vi "projektjki.vi"() -> ()   [LabVIEW 2020]
uses:
  <vilib>/vision/driver/NI_Vision_Acquisition_Software.lvlib
panel:
  out "Informacje":string
  out "Wykryto kamere":bool
  out "?":bool
  out "Mało wody":bool
  out "Dużo wody":bool
  out "Kamera aktywna":bool
  out "Zapis danychh":bool
  in  "Zapis danych":bool
  out "cm^3                                     Tank":dbl(slide) scale=0.0..394.0
  in  "Wl/WYL Kamere":bool
  out "Image":T1(plugin-control)
  in  "Zakoncz":bool
  # "Zbiornik"
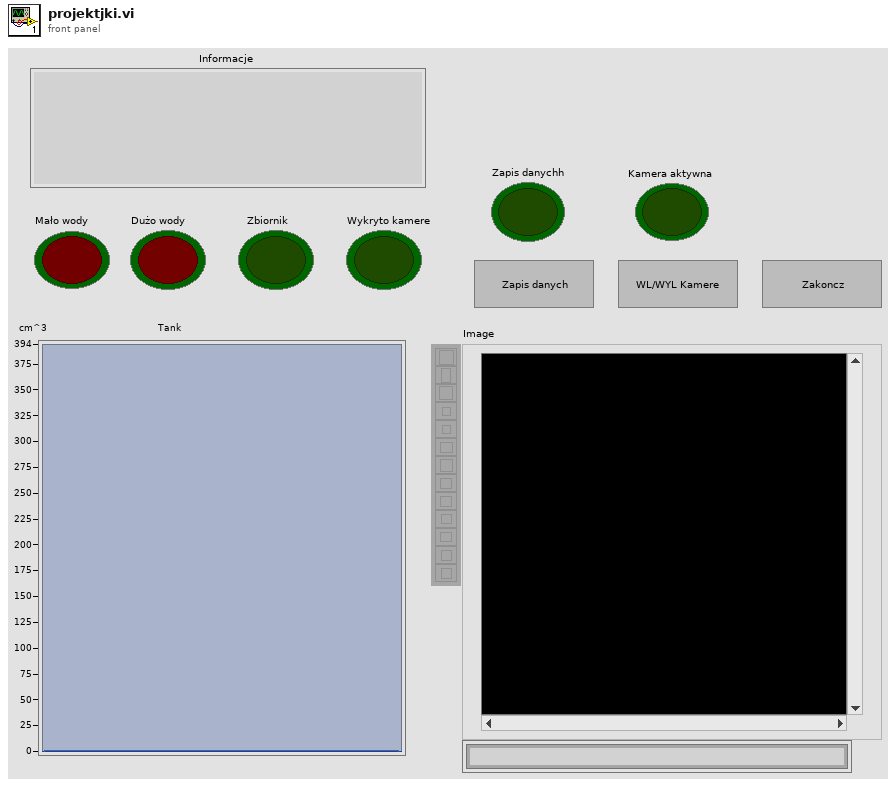
[diagram p1: front panel]
types:
  T1 = typedef "IMAQ Image.ctl" = refnum<image>
  T2 = enum32{"Invalid", "Standard", "Closed", "Hidden", "Minimized", "Maximized"}
  T3 = enum32{"invalid app kind", "Development System", "Run Time System", "Student Edition", "Embedded LabVIEW", "Evaluation", "Custom"}
  T4 = cluster{"Core":cluster{"Current VI Reference":refnum<vi>, "Close Panel on Exit?":bool}, "wykryto kamere":bool, "\nInformacje":string, "Image":T1, "Wylacz kamere":bool, "number of replacements":i32, "historia zbiornika":dbl, "cm^3                                     Tank ":dbl, "Zapis danych":bool, "Mało wody":bool, "Dużo wody":bool, "Wykryto obiekt":bool}
  T5 = cluster{"Current VI Reference":refnum<vi>, "Close Panel on Exit?":bool}
  T6 = cluster{"Point1 (Pixels)":cluster{"X":sgl, "Y":sgl}, "Point2 (Pixels)":cluster{"X":sgl, "Y":sgl}, "Point1 (Real-World)":cluster{"X":sgl, "Y":sgl}, "Point2 (Real-World)":cluster{"X":sgl, "Y":sgl}, "Angle (Pixel)":dbl, "Angle (Real-World)":dbl, "Score":dbl, "Straightness":dbl, "Average SNR (db)":dbl, "Calibration Valid":bool}[]
  T7 = cluster{"Point1 (Pixels)":cluster{"X":sgl, "Y":sgl}, "Point2 (Pixels)":cluster{"X":sgl, "Y":sgl}, "Point1 (Real-World)":cluster{"X":sgl, "Y":sgl}, "Point2 (Real-World)":cluster{"X":sgl, "Y":sgl}, "Angle (Pixel)":dbl, "Angle (Real-World)":dbl, "Score":dbl, "Straightness":dbl, "Average SNR (db)":dbl, "Calibration Valid":bool}
  T8 = cluster{"Type":u32, "Version":u32, "Flags":u32, "SerialNumberHigh":u32, "SerialNumberLow":u32, "BusType":u32, "InterfaceName":string, "VendorName":string, "ModelName":string, "CameraFileName":string, "CameraAttributeURL":string}[]
  T9 = cluster{"Type":u32, "Version":u32, "Flags":u32, "SerialNumberHigh":u32, "SerialNumberLow":u32, "BusType":u32, "InterfaceName":string, "VendorName":string, "ModelName":string, "CameraFileName":string, "CameraAttributeURL":string}
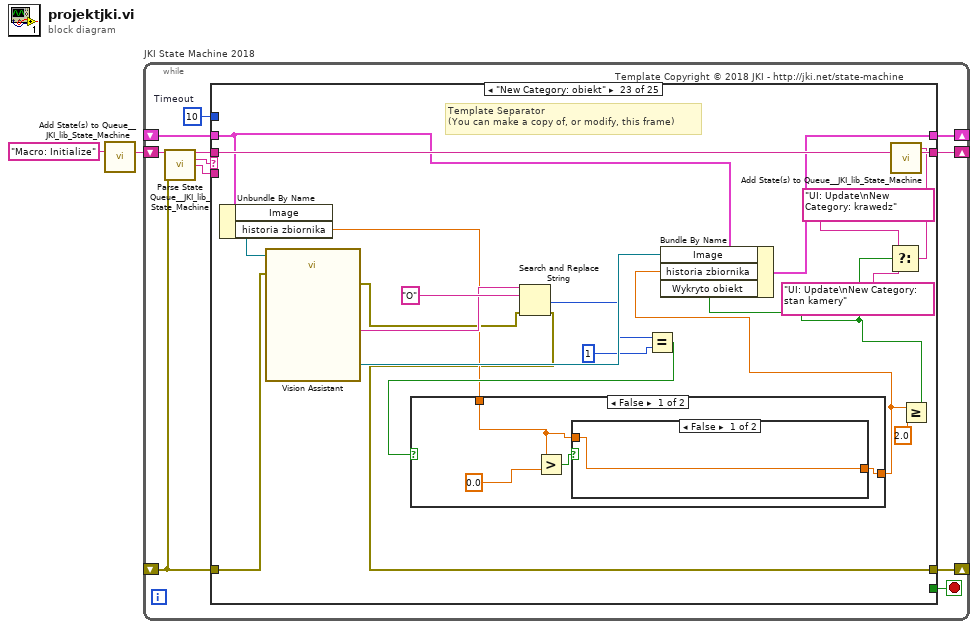
[diagram p0: block diagram]
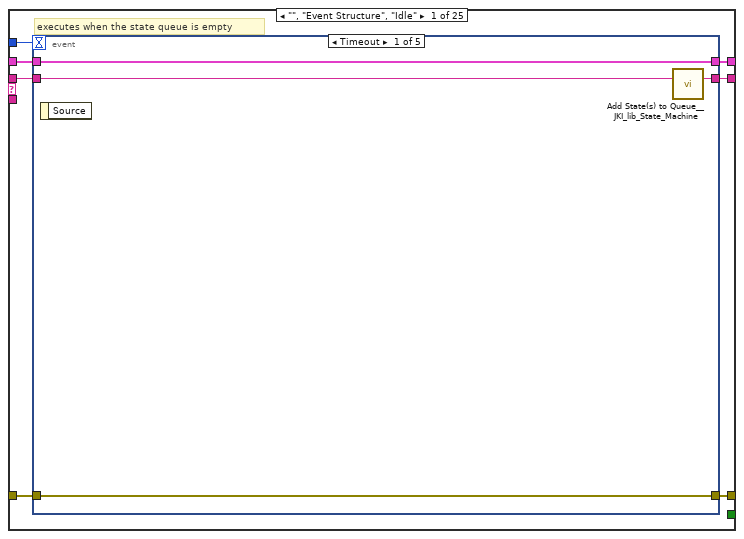
[diagram p2: hidden frame]
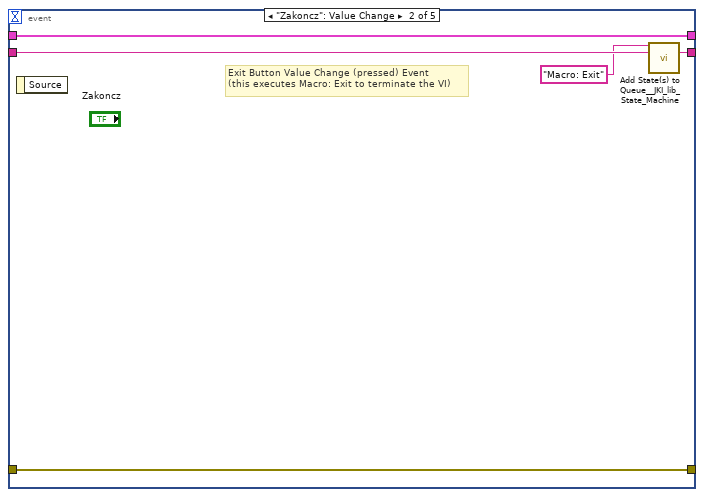
[diagram p3: hidden frame]
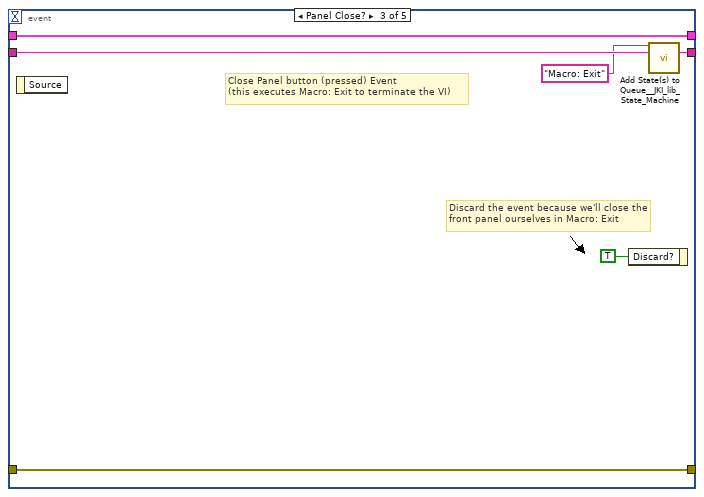
[diagram p4: hidden frame]
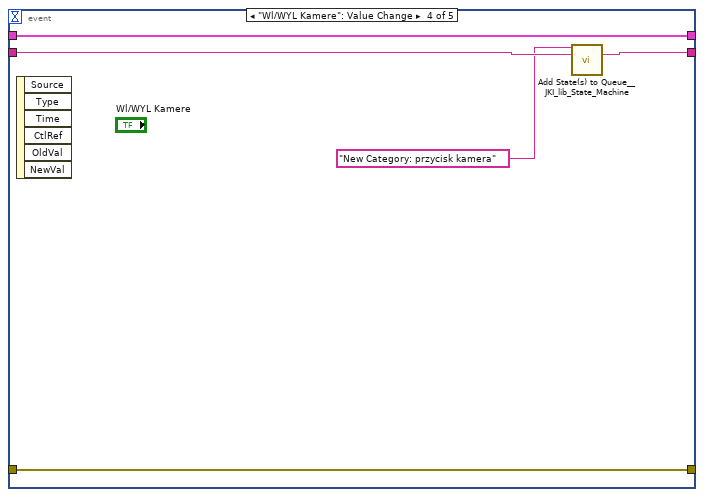
[diagram p5: hidden frame]
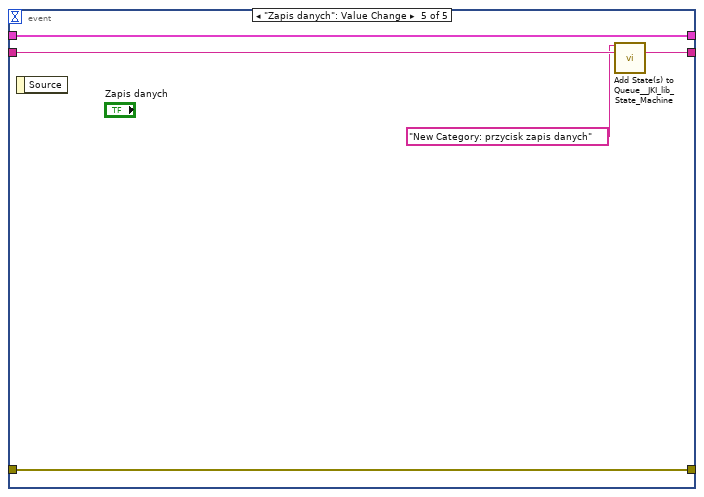
[diagram p6: hidden frame]
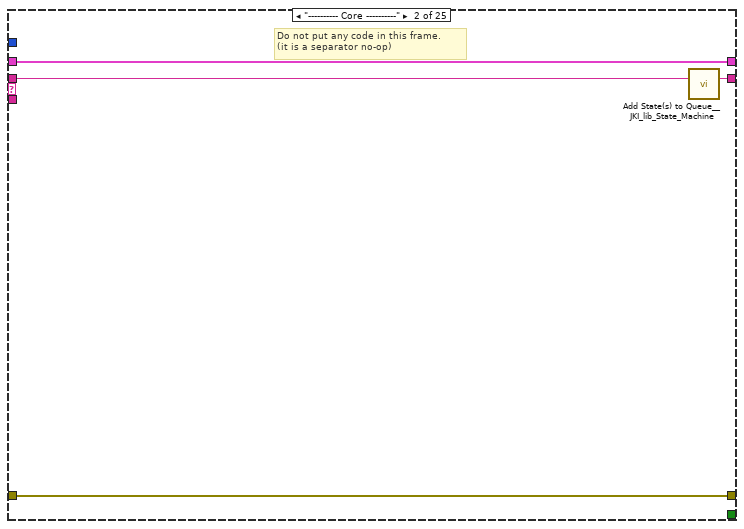
[diagram p7: hidden frame]
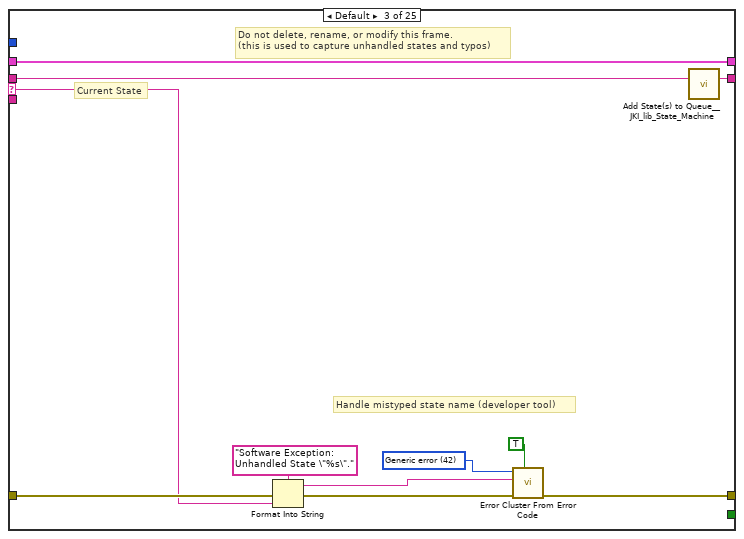
[diagram p8: hidden frame]
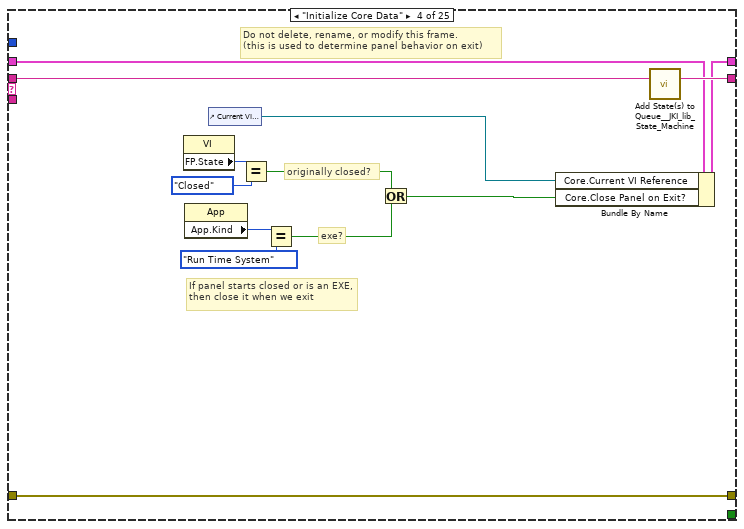
[diagram p9: hidden frame]
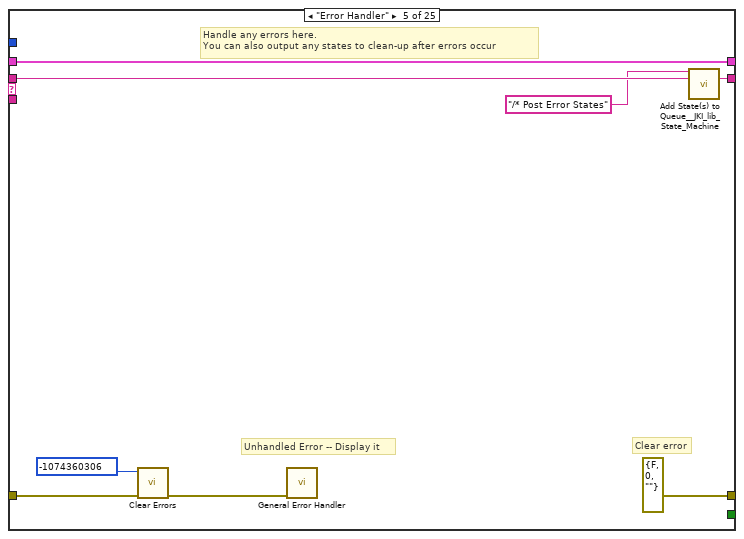
[diagram p10: hidden frame]
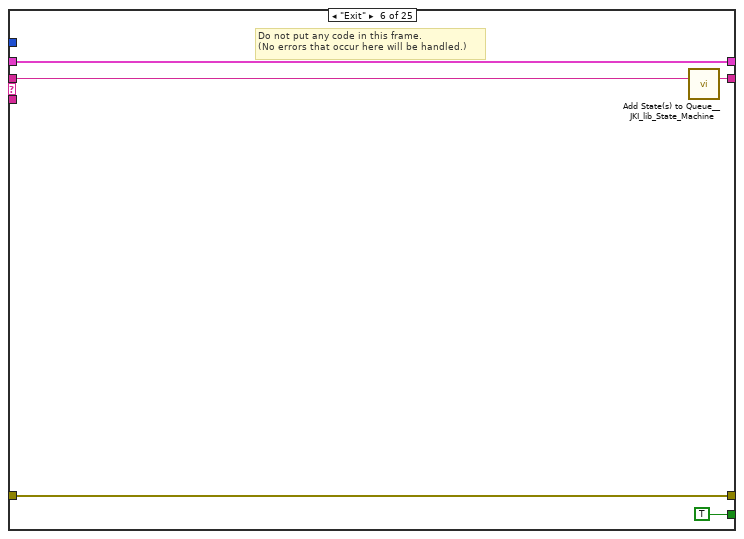
[diagram p11: hidden frame]
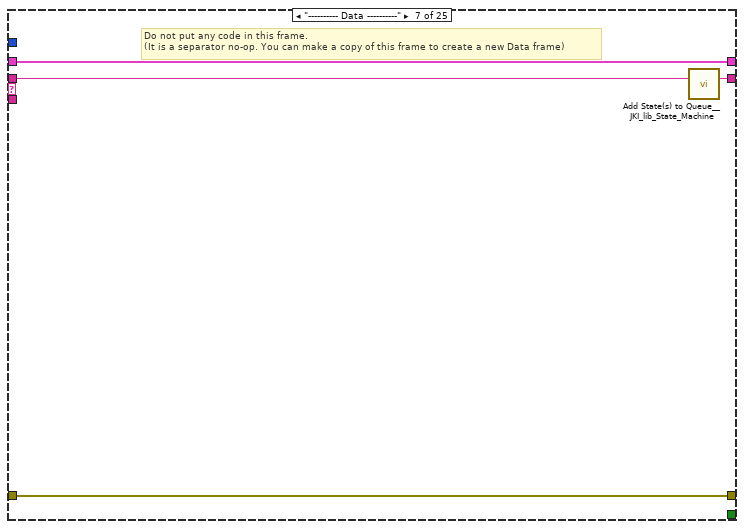
[diagram p12: hidden frame]
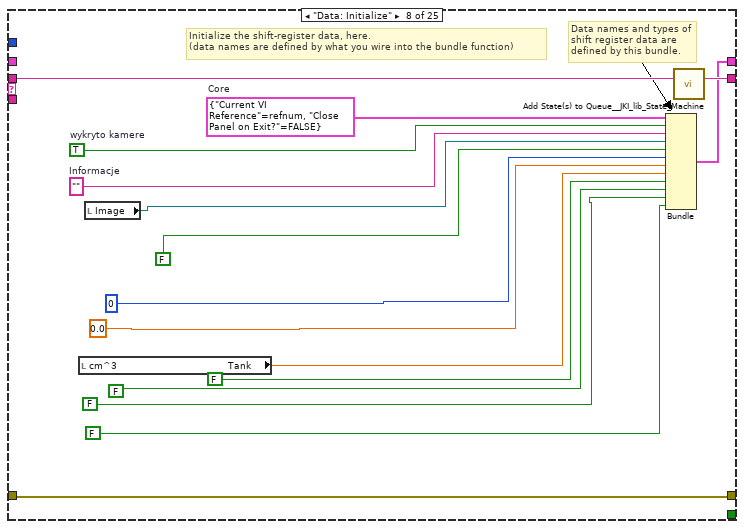
[diagram p13: hidden frame]
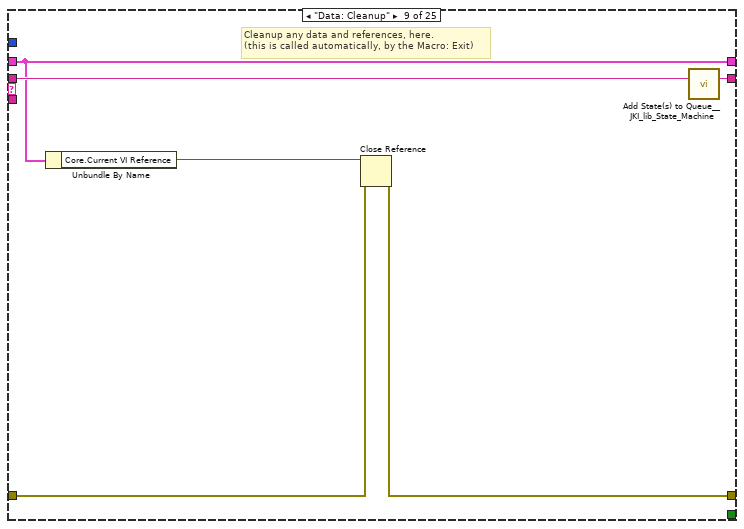
[diagram p14: hidden frame]
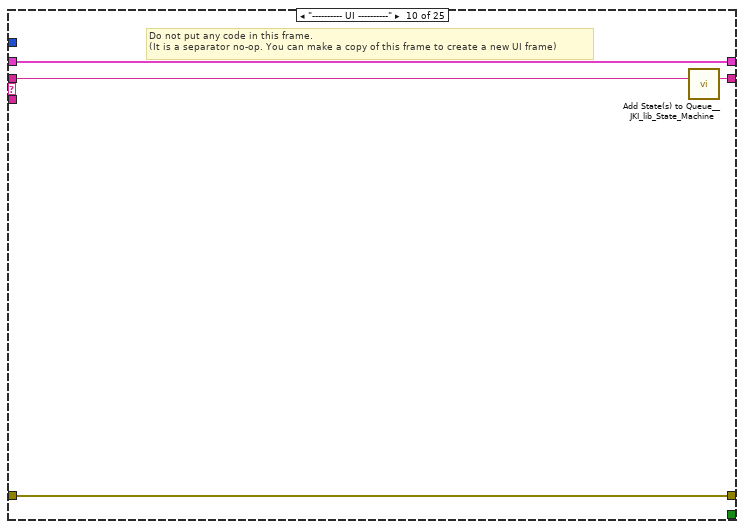
[diagram p15: hidden frame]
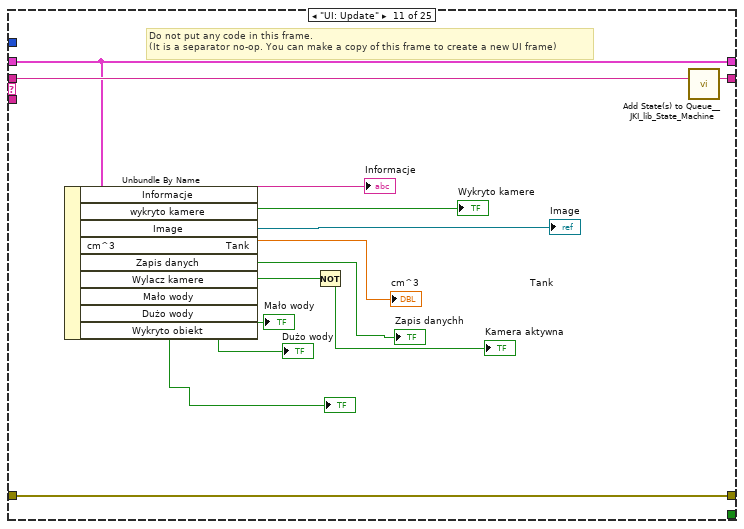
[diagram p16: hidden frame]
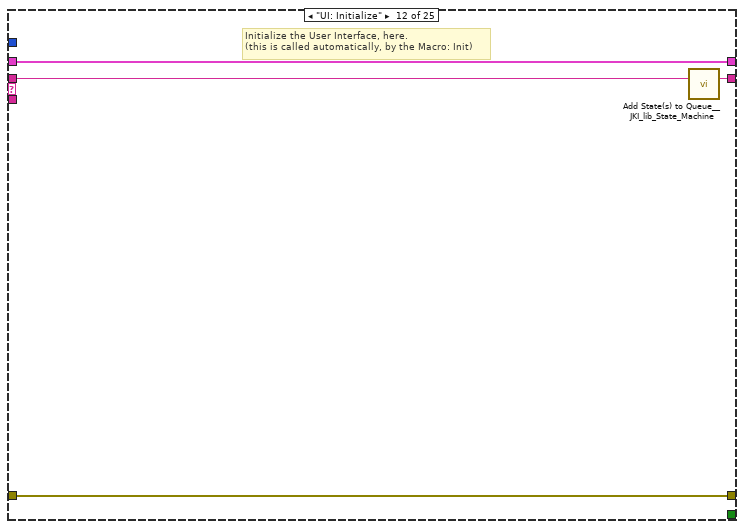
[diagram p17: hidden frame]
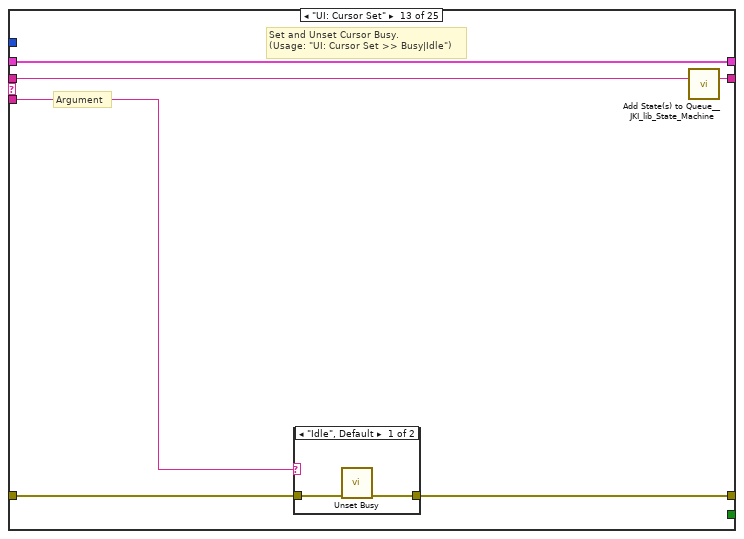
[diagram p18: hidden frame]
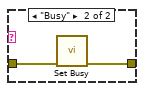
[diagram p19: hidden frame]
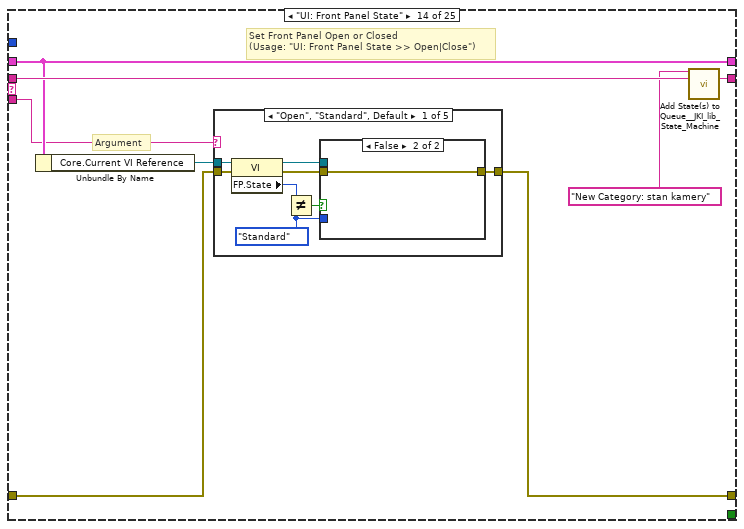
[diagram p20: hidden frame]
diagram:
  n1 = call <vilib>:"Add State(s) to Queue__JKI_lib_State_Machine.vi"("State(s) in (\"\")"="Macro: Initialize") -> ("States Out"=w2:string)  [unwired: 14 in]
  n2 = while "JKI State Machine 2018" {
    shift-right: [w6] -> _
    shift-left: _ -> [w5]
    shift-right: [w9] -> _
    shift-left: _ -> [w3]
    shift-right: [w8] -> _
    shift-left: w2 -> [w10]
    stop <- w7 stop-if-true
    w4 = 10  # Timeout
    # "Template Copyright © 2018 JKI - http://jki.net/state-machine"
    n3 = call <vilib>:"Parse State Queue__JKI_lib_State_Machine.vi"("State Queue"=w10, "Error In (no error)"=w3) -> ("Remaining States"=w12:string, "Current State"=w13:string, "Arguments"=w11:string)  [unwired: 11 in]
    n4 = case shown="\"New Category: obiekt\"" w13 {
      selector: w13 -> [_ _ w50 _ _ _ _ _ _ _ _ _ _ _ _ _ _ _ _ _ _ _ _ _ _]
      tunnel: w12 -> [w20 w49 w54 w73 w81 w86 w90 w106 w112 w116 w130 w134 w140 w152 w221 w231 w236 w240 w250 w257 w270 w288 w324 w353 w374]
      tunnel: w11 -> [_ _ _ _ _ _ _ _ _ _ _ _ w135 w146 _ _ _ _ _ _ _ _ _ _ _]
      tunnel: w5 -> [w18 w46 w52 w66 w78 w84 w87 _ w107 w113 w127 w132 w138 w148 w218 w228 w233 w237 w247 w253 w260 w280 w320 w349 w360]
      tunnel: [w17 w47 w56 w70 errorcluster {"status"=FALSE, "code"=0, "source"=""} ("error out") w83 w88 w103 w108 w114 w128 w131 w136 w149 w219 w229 w234 w238 w248 w255 w265 w278 w304 w341 w371] -> w9
      tunnel: w3 -> [w16 w47 w55 w70 w74 w83 w88 w103 w109 w114 w128 w131 w137 w150 w219 w229 w234 w238 w248 w255 w264 w277 w307 w343 w370]
      tunnel: [w19 w48 w53 w72 w80 w85 w89 w105 w111 w115 w129 w133 w139 w151 w220 w230 w235 w239 w249 w256 w269 w287 w323 w352 w373] -> w8
      tunnel: [_ _ _ _ _ TRUE _ _ _ _ _ _ _ _ _ _ _ _ _ _ _ _ _ _ _] -> w7
      tunnel: [w15 w46 w52 w71 w78 w84 w87 w104 w107 w113 w127 w132 w138 w148 w218 w228 w233 w237 w243 w254 w261 w281 w321 w351 w361] -> w6
      tunnel: w4 -> [w14 _ _ _ _ _ _ _ _ _ _ _ _ _ _ _ _ _ _ _ _ _ _ _ _]
      frame "", "Event Structure", "Idle" {
        # "executes when the state queue is empty"
        n5 = event shown="[0] Timeout" {
          selector: _ -> [_ _ _ _ _]
          dyn-events: _ -> [_ _ _ _ _]
          timeout: w14 -> [_ _ _ _ _]
          tunnel: w20 -> [w24 w29 w35 w37 w43]
          tunnel: [w23 w28 w34 w38 w44] -> w19
          tunnel: w18 -> [w21 w26 w32 w40 w45]
          tunnel: [w22 w27 w33 w39 w41] -> w17
          tunnel: w16 -> [w22 w27 w33 w39 w41]
          tunnel: [w21 w26 w32 w40 w45] -> w15
          event Timeout {
            n6 = event-data() -> ()  [unwired: 1 in, 1 out]
            n7 = call <vilib>:"Add State(s) to Queue__JKI_lib_State_Machine.vi"("State(s) in (\"\")"=w24) -> ("States Out"=w23:string)  [unwired: 14 in]
          }
          event "Zakoncz": Value Change {
            # "Exit Button Value Change (pressed) Event\n(this executes Macro: Exit to terminate the VI)"
            n8 = event-data() -> ()  [unwired: 1 in, 1 out]
            n9 = call <vilib>:"Add State(s) to Queue__JKI_lib_State_Machine.vi"("State(s) in Front (\"\")"="Macro: Exit", "State(s) in (\"\")"=w29) -> ("States Out"=w28:string)  [unwired: 13 in]
          }
          event Panel Close? {
            # "Discard the event because we'll close the front panel ourselves in Macro: Exit"
            # "Close Panel button (pressed) Event\n(this executes Macro: Exit to terminate the VI)"
            n10 = event-data() -> ()  [unwired: 1 in, 1 out]
            n11 = event-data ("Event Filter Node")("Discard?"=TRUE) -> ()  [unwired: 1 in, 1 out]
            n12 = call <vilib>:"Add State(s) to Queue__JKI_lib_State_Machine.vi"("State(s) in Front (\"\")"="Macro: Exit", "State(s) in (\"\")"=w35) -> ("States Out"=w34:string)  [unwired: 13 in]
          }
          event "Wl/WYL Kamere": Value Change {
            n13 = event-data() -> ()  [unwired: 1 in, 6 out]
            n14 = call <vilib>:"Add State(s) to Queue__JKI_lib_State_Machine.vi"("State(s) in Front (\"\")"="New Category: przycisk kamera" ("State(s) in Front (\"\")"), "State(s) in (\"\")"=w37) -> ("States Out"=w38:string)  [unwired: 13 in]
          }
          event "Zapis danych": Value Change {
            n15 = event-data() -> ()  [unwired: 1 in, 1 out]
            n16 = call <vilib>:"Add State(s) to Queue__JKI_lib_State_Machine.vi"("State(s) in Front (\"\")"="New Category: przycisk zapis danych" ("State(s) in Front (\"\")"), "State(s) in (\"\")"=w43) -> ("States Out"=w44:string)  [unwired: 13 in]
          }
        }
      }
      frame "---------- Core ----------" {
        # "Do not put any code in this frame.\n(it is a separator no-op)"
        n17 = call <vilib>:"Add State(s) to Queue__JKI_lib_State_Machine.vi"("State(s) in (\"\")"=w49) -> ("States Out"=w48:string)  [unwired: 14 in]
      }
      frame Default {
        w59 = 42 items=["No error", "Argument error", "Memory is full", "Out of zone", "End of file", "File already open", "Generic file I/O error", "File not found", "File permission error", "Disk is full", "Duplicate path", "Too many files open", "System feature not enabled", "Resource file not found", "Cannot add resource", "Resource not found", "Image not found", "Image memory error", "Pen does not exist", "Config type invalid", "Config token not found", "Config parse error", "Config memory error", "Bad external code format", "Bad external code offset", "External code not present", "Null window", "Destroy window error", "Null menu", "Print aborted", "Bad print record", "Print driver error", "Windows error during printing", "Memory error during printing", "Print dialog error", "Generic print error", "Invalid device refnum", "Device not found", "Device parameter error", "Device unit error", "Cannot open device", "Device call aborted", "Generic error", "Cancelled by user", "Object ID too low", "Object ID too high", "Object not in heap", "Unknown heap", "Unknown object (invalid DefProc)", "Unknown object (DefProc not in table)", "Message out of range", "Invalid (null) method", "Unknown message", "Manager call not supported", "Bad address", "Network operation in progress", "Network operation timed out", "Connection is busy", "Network attribute not supported", "Network error", "Address in use", "System out of memory", "Connection aborted", "Connection refused", "Not connected", "Already connected", "Connection closed", "Initialization error (interapplication manager)", "Bad occurrence", "Wait on unbound occurrence handler", "Occurrence queue overflow", "Datalog type conflict", "Unused", "Unrecognized type (interapplication manager)", "Memory corrupt", "Failed to make temporary DLL", "Old CIN version", "Drag socket not found", "Failed to load drop-object", "Failed to register OLE object", "Failed to release OLE object", "Format specifier type mismatch", "Unknown format specifier", "Too few format specifiers", "Too many format specifiers", "Scan failed", "Newer CIN version", "Error converting to variant", "Runtime menu error", "Password tampered", "Variant attribute not found", "Incompatible variant data type", "Event data is not available", "Event Store is not present", "Occurrence is not found", "Event Queue is not created", "Event info is not available", "Refnum passed is NULL", "Error retrieving Class GUID", "Error retrieving CoClass GUID", "Error retrieving TypeLib GUID.", "Bad built application magic bytes.", "Specific driver is different from the specific driver associated with the Logical Name.", "There is no session opened to the class driver.", "Max Error", "MAX - Error with config objects", "MAX - Error loading configuration", "MAX - Group not supported"]
        # "Current State"
        # "Do not delete, rename, or modify this frame.\n(this is used to capture unhandled states and typos)"
        # "Handle mistyped state name (developer tool)"
        n18 = Format Into String(format string="Software Exception: Unhandled State \"%s\"." ("message"), error in=w55, w50) -> (resulting string=w58:string, error out=w57:errorcluster)  [unwired: 1 in]
        n19 = call <vilib>:"Error Cluster From Error Code.vi"("show call chain? (False)"=TRUE, "error in (no error)"=w57, "error message (\"\")"=w58, "error code (0)"=w59) -> ("error out"=w56:errorcluster)  [unwired: 5 in]
        n20 = call <vilib>:"Add State(s) to Queue__JKI_lib_State_Machine.vi"("State(s) in (\"\")"=w54) -> ("States Out"=w53:string)  [unwired: 14 in]
      }
      frame "Initialize Core Data" {
        # "Do not delete, rename, or modify this frame.\n(this is used to determine panel behavior on exit)"
        # "originally closed?"
        # "exe?"
        # "If panel starts closed or is an EXE, then close it when we exit"
        n21 = property on="Property Node" class="VI"() -> ("FP.State"=w63:T2)  [unwired: 2 in, 2 out]
        n22 = property on="Property Node" class="App"() -> ("App.Kind"=w69:T3)  [unwired: 2 in, 2 out]
        n23 = control-ref of="Current VI Reference"() -> (w64:refnum<vi>)
        n24 = Equal?(x=w63, y=T2."Closed" ("Front Panel Window:State")) -> (x = y?=w61:bool)
        n25 = Equal?(x=w69, y=T3."Run Time System" ("Application:Kind")) -> (x = y?=w67:bool)
        n26 = Or(x=w61, y=w67) -> (x .or. y?=w65:bool)
        n27 = Bundle By Name(cluster=w66, "Core.Current VI Reference"=w64, "Core.Close Panel on Exit?"=w65) -> (w71:T4)
        n28 = call <vilib>:"Add State(s) to Queue__JKI_lib_State_Machine.vi"("State(s) in (\"\")"=w73) -> ("States Out"=w72:string)  [unwired: 14 in]
      }
      frame "Error Handler" {
        # "Unhandled Error -- Display it"
        # "Handle any errors here.\nYou can also output any states to clean-up after errors occur"
        # "Clear error"
        n29 = call <vilib>:"Clear Errors.vi"("error in (no error)"=w74, "specific error code to clear (0: all)"=-1074360306) -> ("error out"=w75:errorcluster)  [unwired: 4 in, 1 out]
        n30 = call <vilib>:"General Error Handler.vi"("error in (no error)"=w75) -> ()  [unwired: 10 in, 5 out]
        n31 = call <vilib>:"Add State(s) to Queue__JKI_lib_State_Machine.vi"("State(s) in Front (\"\")"="/* Post Error States", "State(s) in (\"\")"=w81) -> ("States Out"=w80:string)  [unwired: 13 in]
      }
      frame "Exit" {
        # "Do not put any code in this frame.\n(No errors that occur here will be handled.)"
        n32 = call <vilib>:"Add State(s) to Queue__JKI_lib_State_Machine.vi"("State(s) in (\"\")"=w86) -> ("States Out"=w85:string)  [unwired: 14 in]
      }
      frame "---------- Data ----------" {
        # "Do not put any code in this frame.\n(It is a separator no-op. You can make a copy of this frame to create a new Data frame)"
        n33 = call <vilib>:"Add State(s) to Queue__JKI_lib_State_Machine.vi"("State(s) in (\"\")"=w90) -> ("States Out"=w89:string)  [unwired: 14 in]
      }
      frame "Data: Initialize" {
        w100 = T5 {"Current VI Reference"=refnum, "Close Panel on Exit?"=FALSE}  # Core
        w102 = TRUE  # wykryto kamere
        w101 = ""  # Informacje
        # "Data names and types of shift register data are defined by this bundle."
        # "Initialize the shift-register data, here.\n(data names are defined by what you wire into the bundle function)"
        n34 = local read "cm^3                                     Tank"() -> (w98:dbl)
        n35 = local read "Image"() -> (w91:T1)
        n36 = Bundle("Core"=w100, "wykryto kamere"=w102, "Informacje"=w101, "Image"=w91, "Wylacz kamere"=FALSE, "number of replacements"=0, "historia zbiornika"=0.0, "cm^3                                     Tank"=w98, "Zapis danych"=FALSE, "Mało wody"=FALSE, "Dużo wody"=FALSE, "Wykryto obiekt"=FALSE) -> (w104:T4)  [unwired: 1 in]
        n37 = call <vilib>:"Add State(s) to Queue__JKI_lib_State_Machine.vi"("State(s) in (\"\")"=w106) -> ("States Out"=w105:string)  [unwired: 14 in]
      }
      frame "Data: Cleanup" {
        # "Cleanup any data and references, here.\n(this is called automatically, by the Macro: Exit)"
        n38 = Unbundle By Name(w107) -> ("Core.Current VI Reference"=w110:refnum<vi>)
        n39 = Close Reference(reference=w110, error in (no error)=w109) -> (error out=w108:errorcluster)
        n40 = call <vilib>:"Add State(s) to Queue__JKI_lib_State_Machine.vi"("State(s) in (\"\")"=w112) -> ("States Out"=w111:string)  [unwired: 14 in]
      }
      frame "---------- UI ----------" {
        # "Do not put any code in this frame.\n(It is a separator no-op. You can make a copy of this frame to create a new UI frame)"
        n41 = call <vilib>:"Add State(s) to Queue__JKI_lib_State_Machine.vi"("State(s) in (\"\")"=w116) -> ("States Out"=w115:string)  [unwired: 14 in]
      }
      frame "UI: Update" {
        # "Do not put any code in this frame.\n(It is a separator no-op. You can make a copy of this frame to create a new UI frame)"
        n42 = Unbundle By Name(w127) -> ("Informacje"=→"Informacje":string, "wykryto kamere"=→"Wykryto kamere":bool, "Image"=→"Image":T1, "cm^3                                     Tank"=→"cm^3                                     Tank":dbl, "Zapis danych"=→"Zapis danychh":bool, "Wylacz kamere"=w123:bool, "Mało wody"=→"Mało wody":bool, "Dużo wody"=→"Dużo wody":bool, "Wykryto obiekt"=→"?":bool)
        n43 = Not(x=w123) -> (.not. x?=→"Kamera aktywna":bool)
        n44 = call <vilib>:"Add State(s) to Queue__JKI_lib_State_Machine.vi"("State(s) in (\"\")"=w130) -> ("States Out"=w129:string)  [unwired: 14 in]
      }
      frame "UI: Initialize" {
        # "Initialize the User Interface, here.\n(this is called automatically, by the Macro: Init)"
        n45 = call <vilib>:"Add State(s) to Queue__JKI_lib_State_Machine.vi"("State(s) in (\"\")"=w134) -> ("States Out"=w133:string)  [unwired: 14 in]
      }
      frame "UI: Cursor Set" {
        # "Argument"
        # "Set and Unset Cursor Busy.\n(Usage: \"UI: Cursor Set >> Busy|Idle\")"
        n46 = case shown="\"Idle\", Default" w135 {
          tunnel: w137 -> [w142 w144]
          tunnel: [w141 w143] -> w136
          frame "Idle", Default {
            n47 = call <vilib>:"Unset Busy.vi"("error in (no error)"=w142) -> ("error out"=w141:errorcluster)  [unwired: 10 in]
          }
          frame "Busy" {
            n48 = call <vilib>:"Set Busy.vi"("error in (no error)"=w144) -> ("error out"=w143:errorcluster)  [unwired: 9 in, 1 out]
          }
        }
        n49 = call <vilib>:"Add State(s) to Queue__JKI_lib_State_Machine.vi"("State(s) in (\"\")"=w140) -> ("States Out"=w139:string)  [unwired: 14 in]
      }
      frame "UI: Front Panel State" {
        # "Argument"
        # "Set Front Panel Open or Closed\n(Usage: \"UI: Front Panel State >> Open|Close\")"
        n50 = Unbundle By Name(w148) -> ("Core.Current VI Reference"=w147:refnum<vi>)
        n51 = case shown="\"Open\", \"Standard\", Default" w146 {
          tunnel: w150 -> [w158 w173 w184 w197 w210]
          tunnel: [w160 w174 w186 w199 w212] -> w149
          tunnel: w147 -> [w159 w171 w185 w198 w211]
          frame "Open", "Standard", Default {
            w153 = T2."Standard" ("State")
            n52 = property on="Property Node" class="VI"(reference=w159, error in=w158) -> (reference out=w156:refnum<vi>, error out=w157:errorcluster, "FP.State"=w155:T2)
            n53 = Not Equal?(x=w155, y=w153) -> (x != y?=w154:bool)
            n54 = case shown="False" w154 {
              tunnel: [w164 w166] -> w160
              tunnel: w157 -> [w163 w166]
              tunnel: w156 -> [w162 _]
              tunnel: w153 -> [w161 _]
              frame True {
                n55 = invoke on="Invoke Node" class="VI" method="FP.Open"(reference=w162, error in=w163, "Activate"=TRUE, "State"=w161) -> (error out=w164:errorcluster)  [unwired: 1 in, 4 out]
              }
              frame False {
              }
            }
          }
          frame "Close", "Closed" {
            n56 = property on="Property Node" class="VI"(reference=w171, error in=w173) -> (reference out=w170:refnum<vi>, error out=w172:errorcluster, "FP.State"=w168:T2)
            n57 = Not Equal?(x=w168, y=T2."Closed" ("Front Panel Window:State")) -> (x != y?=w167:bool)
            n58 = case shown="True" w167 {
              tunnel: [w175 w178] -> w174
              tunnel: w172 -> [w175 w177]
              tunnel: w170 -> [_ w176]
              frame False {
              }
              frame True {
                n59 = invoke on="Invoke Node" class="VI" method="FP.Close"(reference=w176, error in=w177) -> (error out=w178:errorcluster)  [unwired: 1 in, 2 out]
              }
            }
          }
          frame "Hidden", "Hide" {
            w179 = T2."Hidden" ("State")
            n60 = property on="Property Node" class="VI"(reference=w185, error in=w184) -> (reference out=w182:refnum<vi>, error out=w183:errorcluster, "FP.State"=w181:T2)
            n61 = Not Equal?(x=w181, y=w179) -> (x != y?=w180:bool)
            n62 = case shown="True" w180 {
              tunnel: [w190 w191] -> w186
              tunnel: w183 -> [w189 w191]
              tunnel: w182 -> [w188 _]
              tunnel: w179 -> [w187 _]
              frame True {
                n63 = invoke on="Invoke Node" class="VI" method="FP.Open"(reference=w188, error in=w189, "State"=w187) -> (error out=w190:errorcluster)  [unwired: 2 in, 4 out]
              }
              frame False {
              }
            }
          }
          frame "Minimize", "Minimized" {
            w192 = T2."Minimized" ("State")
            n64 = property on="Property Node" class="VI"(reference=w198, error in=w197) -> (reference out=w195:refnum<vi>, error out=w196:errorcluster, "FP.State"=w194:T2)
            n65 = Not Equal?(x=w194, y=w192) -> (x != y?=w193:bool)
            n66 = case shown="True" w193 {
              tunnel: [w203 w204] -> w199
              tunnel: w196 -> [w202 w204]
              tunnel: w195 -> [w201 _]
              tunnel: w192 -> [w200 _]
              frame True {
                n67 = invoke on="Invoke Node" class="VI" method="FP.Open"(reference=w201, error in=w202, "State"=w200) -> (error out=w203:errorcluster)  [unwired: 2 in, 4 out]
              }
              frame False {
              }
            }
          }
          frame "Maximize", "Maximized" {
            w205 = T2."Maximized" ("State")
            n68 = property on="Property Node" class="VI"(reference=w211, error in=w210) -> (reference out=w208:refnum<vi>, error out=w209:errorcluster, "FP.State"=w207:T2)
            n69 = Not Equal?(x=w207, y=w205) -> (x != y?=w206:bool)
            n70 = case shown="True" w206 {
              tunnel: [w216 w217] -> w212
              tunnel: w209 -> [w215 w217]
              tunnel: w208 -> [w214 _]
              tunnel: w205 -> [w213 _]
              frame True {
                n71 = invoke on="Invoke Node" class="VI" method="FP.Open"(reference=w214, error in=w215, "State"=w213) -> (error out=w216:errorcluster)  [unwired: 2 in, 4 out]
              }
              frame False {
              }
            }
          }
        }
        n72 = call <vilib>:"Add State(s) to Queue__JKI_lib_State_Machine.vi"("State(s) in Front (\"\")"="New Category: stan kamery" ("State(s) in Front (\"\")"), "State(s) in (\"\")"=w152) -> ("States Out"=w151:string)  [unwired: 13 in]
      }
      frame "---------- Macro ----------" {
        # "Do not put any code in this frame.\n(It is a separator no-op. You can make a copy of this frame to create a new Macro frame)"
        n73 = call <vilib>:"Add State(s) to Queue__JKI_lib_State_Machine.vi"("State(s) in (\"\")"=w221) -> ("States Out"=w220:string)  [unwired: 14 in]
      }
      frame "Macro: Exit" {
        # "Exit Macro\n(This is called once, when the VI exits)"
        n74 = Unbundle By Name(w228) -> ("Core.Close Panel on Exit?"=w227:bool)
        n75 = Select(t="UI: Front Panel State >> Close", s=w227, f="" ("Empty String Constant")) -> (s? t:f=w224:string)
        n76 = call <vilib>:"Add State(s) to Queue__JKI_lib_State_Machine.vi"("State(s) in (\"\")"=w224, "State(s) at Back (\"\")"="Data: Cleanup\nExit") -> ("States Out"=w222:string)  [unwired: 13 in]
        n77 = call <vilib>:"Add State(s) to Queue__JKI_lib_State_Machine.vi"("State(s) in Front (\"\")"=w222, "State(s) in (\"\")"=w231) -> ("States Out"=w230:string)  [unwired: 13 in]
      }
      frame "Macro: Initialize" {
        w232 = "Data: Initialize\nInitialize Core Data\nUI: Initialize\nUI: Front Panel State >> Open"  # Data: Initialize Initialize Core Data UI: Initialize UI: Front Panel State >> Open
        # "Initialization Macro\n(This is called once, when the VI starts)"
        n78 = call <vilib>:"Add State(s) to Queue__JKI_lib_State_Machine.vi"("State(s) in Front (\"\")"=w232, "State(s) in (\"\")"=w236) -> ("States Out"=w235:string)  [unwired: 13 in]
      }
      frame "---------- New Category ----------" {
        # "Template Separator\n(You can make a copy of, or modify, this frame)"
        n79 = call <vilib>:"Add State(s) to Queue__JKI_lib_State_Machine.vi"("State(s) in (\"\")"=w240) -> ("States Out"=w239:string)  [unwired: 14 in]
      }
      frame "New Category: przycisk kamera" {
        # "Template Separator\n(You can make a copy of, or modify, this frame)"
        n80 = Unbundle By Name(w247) -> ("Wylacz kamere"=w246:bool)
        n81 = Not(x=w246) -> (.not. x?=w242:bool)
        n82 = Bundle By Name(cluster=w247, "Wylacz kamere"=w242) -> (w243:T4)
        n83 = Select(t="UI: Update\nNew Category: stan kamery" ("State(s) in Front (\"\")"), s=w242, f="UI: Update\nNew Category: stan kamery") -> (s? t:f=w245:string)
        n84 = call <vilib>:"Add State(s) to Queue__JKI_lib_State_Machine.vi"("State(s) in Front (\"\")"=w245, "State(s) in (\"\")"=w250) -> ("States Out"=w249:string)  [unwired: 13 in]
      }
      frame "New Category: przycisk zapis danych" {
        # "Template Separator\n(You can make a copy of, or modify, this frame)"
        n85 = Unbundle By Name(w253) -> ("Zapis danych"=w252:bool)
        n86 = Not(x=w252) -> (.not. x?=w251:bool)
        n87 = Bundle By Name(cluster=w253, "Zapis danych"=w251) -> (w254:T4)
        n88 = call <vilib>:"Add State(s) to Queue__JKI_lib_State_Machine.vi"("State(s) in (\"\")"=w257) -> ("States Out"=w256:string)  [unwired: 14 in]
      }
      frame "New Category: zapis danych" {
        # "Template Separator\n(You can make a copy of, or modify, this frame)"
        n89 = Unbundle By Name(w260) -> ("cm^3                                     Tank"=w268:dbl, "Zapis danych"=w266:bool)
        n90 = call "bazy.vi"("error in (no error)"=w264, "Boolean"=w266, "Numeric"=w268) -> ("error out"=w265:errorcluster, "code"=w263:i32)  [unwired: 7 in]
        n91 = Equal?(x=w263, y=-2147287038) -> (x = y?=w259:bool)
        n92 = case shown="True" w259 {
          tunnel: ["" ("Informacje") "Zapis danych niemożliwy!!!!\nSprawdź czy podany plik UDL istnieje lub czy znajduje się w podanej ścieżce." ("Informacje")] -> w258
          frame False {
          }
          frame True {
          }
        }
        n93 = Bundle By Name(cluster=w260, "Informacje"=w258) -> (w261:T4)
        n94 = call <vilib>:"Add State(s) to Queue__JKI_lib_State_Machine.vi"("State(s) in Front (\"\")"="New Category: stan kamery" ("State(s) in Front (\"\")"), "State(s) in (\"\")"=w270) -> ("States Out"=w269:string)  [unwired: 13 in]
      }
      frame "New Category: krawedz" {
        # "Template Separator\n(You can make a copy of, or modify, this frame)"
        n95 = Unbundle By Name(w280) -> ("Image"=w286:T1)
        n96 = call "Vision Assistant2"("Image In"=w286, "error in"=w277) -> ("Straight Edges (Adv. Straight Edge 1)"=w285:T6, "error out"=w278:errorcluster)  [unwired: 23 in, 1 out]
        n97 = Index Array(array=w285, index=0) -> (element=w283:T7)
        n98 = Unbundle By Name(w283) -> ("Point1 (Pixels)"=w282:cluster{"X":sgl, "Y":sgl}, "Calibration Valid"=w274:bool)
        n99 = case shown="True" w274 {
          tunnel: w282 -> [_ w303]
          tunnel: [0.0 w292] -> w279
          tunnel: [FALSE w298] -> w276
          tunnel: [TRUE w297] -> w275
          frame False {
          }
          frame True {
            n100 = Unbundle By Name(w303) -> ("Y"=w301:sgl)
            n101 = Subtract(x=720.0, y=w301) -> (x-y=w296:dbl)
            n102 = Greater?(x=w296, y=550.0) -> (0:w298:bool)
            n103 = Less?(x=w296, y=100.0) -> (x < y?=w297:bool)
            n104 = Divide(x=w296, y=50.0) -> (x/y=w294:dbl)
            n105 = Multiply(x=w294, y=28.0) -> (x*y=w292:dbl)
          }
        }
        n106 = Bundle By Name(cluster=w280, "cm^3                                     Tank"=w279, "Mało wody"=w275, "Dużo wody"=w276) -> (w281:T4)
        n107 = call <vilib>:"Add State(s) to Queue__JKI_lib_State_Machine.vi"("State(s) in Front (\"\")"="UI: Update\nNew Category: zapis danych" ("State(s) in Front (\"\")"), "State(s) in (\"\")"=w288) -> ("States Out"=w287:string)  [unwired: 13 in]
      }
      frame "New Category: obiekt" {
        # "Template Separator\n(You can make a copy of, or modify, this frame)"
        n108 = Unbundle By Name(w320) -> ("Image"=w322:T1, "historia zbiornika"=w313:dbl)
        n109 = call "Vision Assistant"("Image In"=w322, "error in"=w307) -> ("Image Out"=w317:T1, "String (OCR/OCV 2)"=w318:string, "error out"=w305:errorcluster)  [unwired: 22 in, 1 out]
        n110 = Search and Replace String(input string=w318, search string="O", error in=w305) -> (number of replacements=w315:i32, error out=w304:errorcluster)  [unwired: 5 in, 2 out]
        n111 = Equal?(x=w315, y=1) -> (x = y?=w314:bool)
        n112 = case shown="False" w314 {
          tunnel: [w325 w334] -> w308
          tunnel: w313 -> [w326 w333]
          frame False {
            n113 = Greater?(x=w326, y=0.0) -> (0:w327:bool)
            n114 = case shown="False" w327 {
              tunnel: w326 -> [w329 w331]
              tunnel: [w329 w330] -> w325
              frame False {
              }
              frame True {
                n115 = Subtract(x=w331, y=1.0) -> (x-y=w330:dbl)
              }
            }
          }
          frame True {
            n116 = Less?(x=w333, y=3.0) -> (x < y?=w335:bool)
            n117 = case shown="False" w335 {
              tunnel: [w337 w339] -> w334
              tunnel: w333 -> [w337 w338]
              frame False {
              }
              frame True {
                n118 = Add(x=w338, y=1.0) -> (x+y=w339:dbl)
              }
            }
          }
        }
        n119 = Greater Or Equal?(x=w308, y=2.0) -> (x >= y?=w306:bool)
        n120 = Bundle By Name(cluster=w320, "Image"=w317, "historia zbiornika"=w308, "Wykryto obiekt"=w306) -> (w321:T4)
        n121 = Select(t="UI: Update\nNew Category: krawedz" ("search string"), s=w306, f="UI: Update\nNew Category: stan kamery" ("search string")) -> (s? t:f=w309:string)
        n122 = call <vilib>:"Add State(s) to Queue__JKI_lib_State_Machine.vi"("State(s) in Front (\"\")"=w309, "State(s) in (\"\")"=w324) -> ("States Out"=w323:string)  [unwired: 13 in]
      }
      frame "New Category: kamera" {
        # "Your code here.\n(You can make a copy of, or modify, this frame)"
        n123 = Unbundle By Name(w349) -> ("Wylacz kamere"=w348:bool)
        n124 = call "Vision Acquisition"("Stop (F)"=w348, "error in"=w343) -> ("Image Out"=w350:T1, "Stopped"=w347:bool, "error out"=w342:errorcluster)  [unwired: 23 in]
        n125 = call <vilib>:"Clear Errors.vi"("error in (no error)"=w342) -> ("error out"=w341:errorcluster)  [unwired: 5 in, 1 out]
        n126 = Bundle By Name(cluster=w349, "Image"=w350) -> (w351:T4)
        n127 = Select(t="UI: Update", s=w347, f="Event Structure\nUI: Update\nNew Category: obiekt" ("State(s) in Front (\"\")")) -> (s? t:f=w346:string)
        n128 = call <vilib>:"Add State(s) to Queue__JKI_lib_State_Machine.vi"("State(s) in Front (\"\")"=w346, "State(s) in (\"\")"=w353) -> ("States Out"=w352:string)  [unwired: 13 in]
      }
      frame "New Category: stan kamery" {
        # "Template Separator\n(You can make a copy of, or modify, this frame)"
        n129 = call <vilib>:"IMAQdx Enumerate Cameras.vi"("error in"=w370, "Connected Only? (Yes)"=TRUE) -> ("error out"=w371:errorcluster, "Camera Information Array"=w369:T8)  [unwired: 8 in]
        n130 = Index Array(array=w369, index=0) -> (element=w367:T9)
        n131 = Unbundle By Name(w367) -> ("InterfaceName"=w366:string)
        n132 = Unbundle By Name(w360) -> ("Wylacz kamere"=w354:bool)
        n133 = Not(x=w354) -> (.not. x?=w355:bool)
        n134 = Equal?(x=w366, y="cam0") -> (x = y?=w357:bool)
        n135 = And(x=w357, y=w355) -> (x .and. y?=w356:bool)
        n136 = Select(t=w354, s=w357, f=TRUE) -> (s? t:f=w358:bool)
        n137 = Select(t="UI: Update\nNew Category: kamera" ("y"), s=w356, f="Event Structure\nUI: Update\nNew Category: stan kamery " ("y")) -> (s? t:f=w362:string)
        n138 = Bundle By Name(cluster=w360, "wykryto kamere"=w357, "Wylacz kamere"=w358) -> (w361:T4)
        n139 = call <vilib>:"Add State(s) to Queue__JKI_lib_State_Machine.vi"("State(s) in Front (\"\")"=w362, "State(s) in (\"\")"=w374) -> ("States Out"=w373:string)  [unwired: 13 in]
      }
    }
  }
